vi "wyciaganie_bitu.vi"(1 "bit number":u64, 2 "number in":u64) -> (0 "is bit set?":bool)   [LabVIEW 2012]
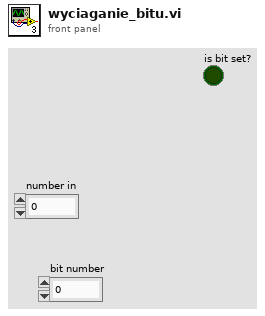
[diagram p1: front panel]
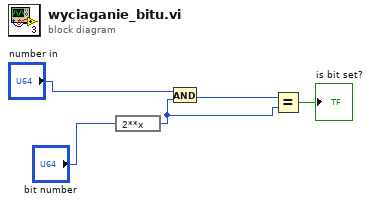
[diagram p0: block diagram]
diagram:
  n1 = expression code="2**x"("bit number") -> (w2:u64)
  n2 = And(x="number in", y=w2) -> (x .and. y?=w3:u64)
  n3 = Equal?(x=w3, y=w2) -> (x = y?=→"is bit set?":bool)
